vi "Read.vi"(8 "error in (no error)":errorcluster caption="entrée d'erreur (pas d'erreur)", 11 "Class UART (Default) en entrée":refnum<class "Class UART (Default).lvclass">) -> (0 "error out":errorcluster caption="sortie d'erreur", 3 "Class UART (Default) en sortie":refnum<class "Class UART (Default).lvclass">)   [LabVIEW 2020, in "Library Instrument & Equipement.lvlib" / "Library UART.lvlib" / "Class UART (Default).lvclass"]
uses:
  Class UART (Default).lvclass
  Class UART (Default).lvclass/Class UART (Default).ctl
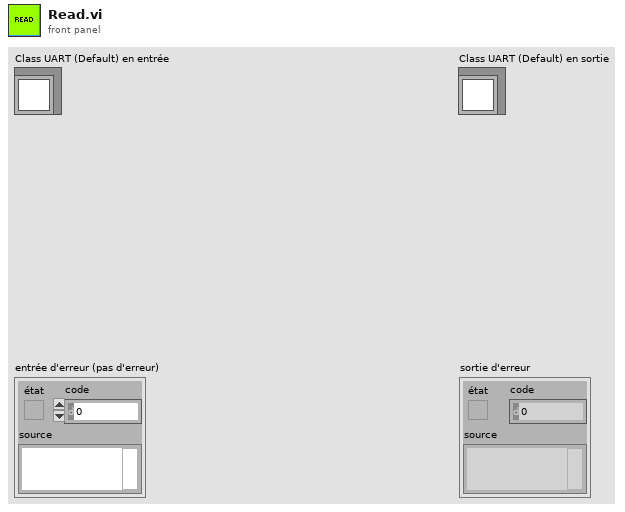
[diagram p1: front panel]
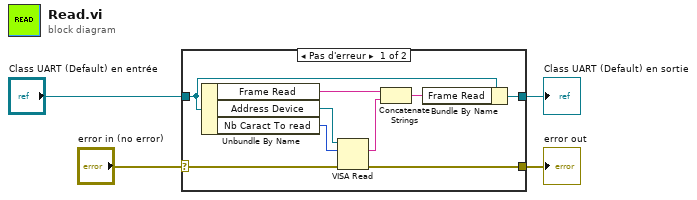
[diagram p0: block diagram]
diagram:
  n1 = case shown="Pas d'erreur" "error in (no error)" {
    selector: "error in (no error)" -> [w12 w15]
    tunnel: [w11 w15] -> w3
    tunnel: [w9 w14] -> w1
    tunnel: "Class UART (Default) en entrée" -> [w10 w14]
    frame No Error {
      n2 = Unbundle By Name(w10) -> ("Frame Read"=w6:string, "Address Device"=w13:refnum<visa-resource-name>, "Nb Caract To read"=w5:u32)
      n3 = VISA Read(VISA resource name=w13, byte count=w5, error in (no error)=w12) -> (read buffer=w8:string, error out=w11:errorcluster)  [unwired: 2 out]
      n4 = Concatenate Strings(w6, w8) -> (w7:string)
      n5 = Bundle By Name(cluster=w10, "Frame Read"=w7) -> (w9:refnum<class "Class UART (Default).lvclass">)
    }
    frame Error {
    }
  }
  "error out" <- w3
  "Class UART (Default) en sortie" <- w1
